vi "Initialise.vi"(6 "Filename":string, 7 "Header":string, 8 "error in (no error)":errorcluster, 9 "Max Records":i32, 10 "Directory":path, 11 "Log in":refnum<class "Log.lvclass">) -> (0 "error out":errorcluster, 3 "Log out":refnum<class "Log.lvclass">)   [LabVIEW 2020, in "RTAF.lvlib" / "Log.lvclass"]
doc: "Sets up the class to beging logging.\n\nThe input file path is checked and all the necessary directories in the chain are created.\n\nThis VI also writes the header to the file."
uses:
  Log.lvclass
  Log.lvclass/Log.ctl
  RTAF.lvlib
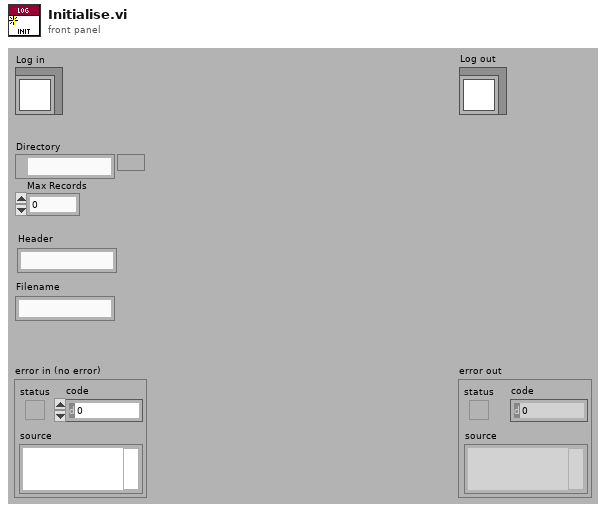
[diagram p1: front panel]
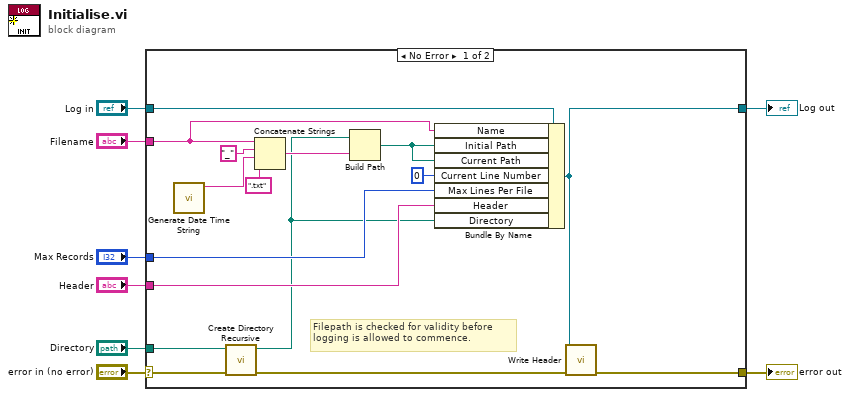
[diagram p0: block diagram]
diagram:
  n1 = case shown="No Error" "error in (no error)" {
    selector: "error in (no error)" -> [w10 w25]
    tunnel: [w21 w25] -> w7
    tunnel: [w13 _] -> w6
    tunnel: "Directory" -> [w11 _]
    tunnel: "Log in" -> [w23 _]
    tunnel: "Max Records" -> [w22 _]
    tunnel: "Header" -> [w20 _]
    tunnel: "Filename" -> [w14 _]
    frame No Error {
      # "Filepath is checked for validity before logging is allowed to commence."
      n2 = call "Generate Date Time String.vi"() -> ("Date time string"=w15:string)  [unwired: 10 in, 1 out]
      n3 = call <vilib>:"Create Directory Recursive.vi"("error in (no error)"=w10, "directory"=w11) -> ("error out"=w9:errorcluster, "directory copy"=w12:path)  [unwired: 3 in, 1 out]
      n4 = Concatenate Strings(w14, "_" ("string"), w15, ".txt" ("string")) -> (w18:string)
      n5 = Build Path(base path=w12, name or relative path=w18) -> (appended path=w17:path)
      n6 = Bundle By Name(cluster=w23, "Name"=w14, "Initial Path"=w17, "Current Path"=w17, "Current Line Number"=0 ("Current Row"), "Max Lines Per File"=w22, "Header"=w20, "Directory"=w12) -> (w13:refnum<class "Log.lvclass">)
      n7 = call "Write Header.vi"("error in (no error)"=w9, "Log in"=w13) -> ("error out"=w21:errorcluster)  [unwired: 1 in, 8 out]
    }
    frame Error {
    }
  }
  "error out" <- w7
  "Log out" <- w6
